vi "Set Ignition Data.vi"(8 "error in":errorcluster, 9 "result_ready":bool, 11 "Ignition in":refnum<class "Ignition.lvclass">) -> (0 "error out":errorcluster, 3 "Ignition out":refnum<class "Ignition.lvclass">)   [LabVIEW 2021, in "Ignition.lvclass"]
uses:
  Ignition.lvclass
  C:/GitHub/OOP_Submodule EOL/Sequence/CodeModules/OPC UA/OPC UA.lvclass
  OPC UA/OPC UA.lvclass/OPC UA.ctl
  Ignition.lvclass/Ignition.ctl
  <vilib>/addons/TestStand/_TSUtility.llb/TestStand - Get Property Value (Number {Signed 32-bit Integer}).vi
  <vilib>/addons/TestStand/_TSUtility.llb/TestStand - Get Property Value (String).vi
  <vilib>/addons/TestStand/_TSUtility.llb/TestStand - Get Property Value (Number {Unsigned 32-bit Integer}).vi
  <vilib>/addons/TestStand/_TSUtility.llb/TestStand - Get Property Value (Numeric Array).vi
  OPC UA/OPC UA.lvclass
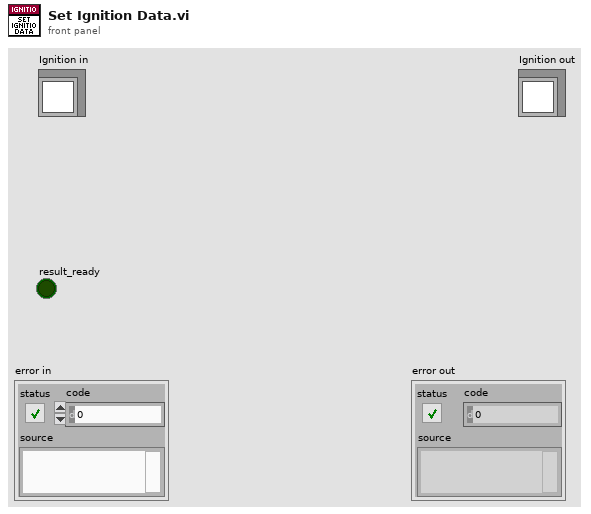
[diagram p1: front panel]
types:
  T1 = typedef "Ignition.lvclass/Tester Tx.ctl" = cluster{"thermistor":dbl, "phase_angle":dbl, "pallet_rfid":dbl, "ocv":dbl, "cell_vsense1":dbl, "cell_vsense2":dbl, "hipot1_leakage_current":dbl, "hipot2_leakage_current":dbl, "guid":string, "can_sn":string, "can_pn":string, "ac_internal_resistance":dbl, "sub_station":string, "fault_code":i32, "elapsed_time":i32, "result":i32, "reject_code_reason":string, "result_ready":bool, "Timeout":bool}
  T2 = cluster{"FaultCode":i32, "Fault codes":cluster{"Bit":string, "Description":string}[]}
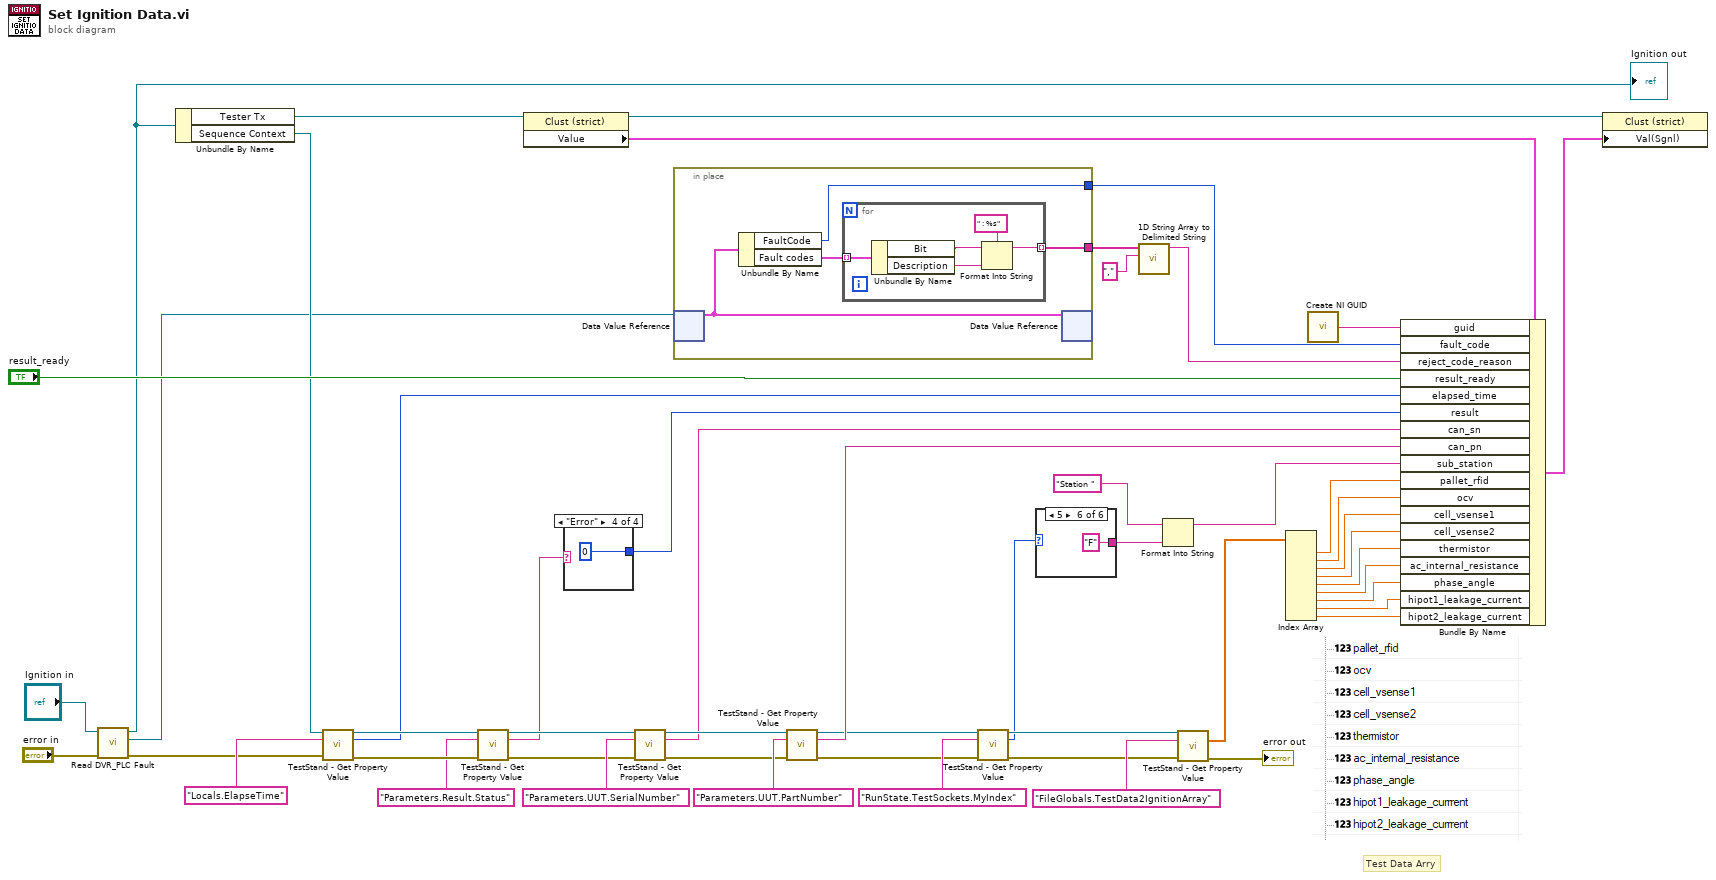
[diagram p0: block diagram]
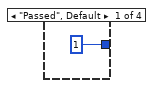
[diagram p2: hidden frame]
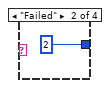
[diagram p3: hidden frame]
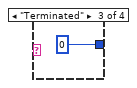
[diagram p4: hidden frame]
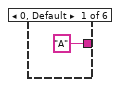
[diagram p5: hidden frame]
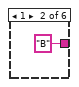
[diagram p6: hidden frame]
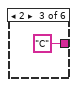
[diagram p7: hidden frame]
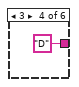
[diagram p8: hidden frame]
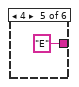
[diagram p9: hidden frame]
diagram:
  # "Test Data Arry"
  n1 = call "Read DVR_PLC Fault.vi"("error in (no error)"="error in", "OPC UA in"="Ignition in") -> ("error out"=w4:errorcluster, "DVR_PLC Fault"=w1:refnum<data-value>, "OPC UA out"=w2:refnum<class "Ignition.lvclass">)  [unwired: 7 in]
  "Ignition out" <- w2
  n2 = Unbundle By Name(w2) -> ("Tester Tx"=w13:refnum<vi>, "Sequence Context"=w14:refnum<k7>)
  n3 = call-poly <vilib>:"TestStand - Get Property Value.vi"("Sequence Context In"=w14, "Lookup String"="Locals.ElapseTime", "error in (no error)"=w4) -> ("Sequence Context Out"=w21:refnum<k7>, "Value"=w17:i32, "error out"=w23:errorcluster)  [unwired: 10 in]
  n4 = call-poly <vilib>:"TestStand - Get Property Value.vi"("Sequence Context In"=w21, "Lookup String"="Parameters.Result.Status", "error in (no error)"=w23) -> ("Sequence Context Out"=w20:refnum<k7>, "Value"=w16:string, "error out"=w19:errorcluster)  [unwired: 10 in]
  n5 = property class="Clust (strict)"(reference=w13) -> (reference out=w11:refnum<vi>, "Value"=w12:T1)  [unwired: 1 in, 1 out]
  n6 = case shown="\"Error\"" w16 {
    tunnel: [1 2 0 0] -> w15
    frame "Passed", Default {
    }
    frame "Failed" {
    }
    frame "Terminated" {
    }
    frame "Error" {
    }
  }
  n7 = call-poly <vilib>:"TestStand - Get Property Value.vi"("Sequence Context In"=w20, "Lookup String"="Parameters.UUT.SerialNumber", "error in (no error)"=w19) -> ("Sequence Context Out"=w51:refnum<k7>, "Value"=w48:string, "error out"=w49:errorcluster)  [unwired: 10 in]
  n8 = in-place {
    in-place-border: [w60] -> w9
    in-place-border: [w58] -> w6
    n9 = in-place-dvr #1(w1) -> (w59:T2)  [unwired: 1 out]
    n10 = Unbundle By Name(w59) -> ("FaultCode"=w58:i32, "Fault codes"=w57:cluster{"Bit":string, "Description":string}[])
    n11 = for {
      tunnel: w57 -> [w63] mode=indexing
      tunnel: [w64] -> w60 mode=indexing
      n12 = Unbundle By Name(w63) -> ("Bit"=w61:string, "Description"=w62:string)
      n13 = Format Into String(format string=" : %s", initial string=w61, w62) -> (resulting string=w64:string)  [unwired: 1 in, 1 out]
    }
    n14 = in-place-dvr #1(w59) -> ()  [unwired: 2 out]
  }
  n15 = call-poly <vilib>:"TestStand - Get Property Value.vi"("Sequence Context In"=w51, "Lookup String"="Parameters.UUT.PartNumber", "error in (no error)"=w49) -> ("Sequence Context Out"=w28:refnum<k7>, "Value"=w47:string, "error out"=w45:errorcluster)  [unwired: 10 in]
  n16 = call-poly <vilib>:"TestStand - Get Property Value.vi"("Sequence Context In"=w28, "Lookup String"="RunState.TestSockets.MyIndex", "error in (no error)"=w45) -> ("Sequence Context Out"=w43:refnum<k7>, "Value"=w27:u32, "error out"=w41:errorcluster)  [unwired: 10 in]
  n17 = case shown="5" w27 {
    tunnel: ["A" ("format string") "B" ("format string") "C" ("format string") "D" ("format string") "E" ("format string") "F" ("format string")] -> w26
    frame 0, Default {
    }
    frame 1 {
    }
    frame 2 {
    }
    frame 3 {
    }
    frame 4 {
    }
    frame 5 {
    }
  }
  n18 = call <vilib>:"1D String Array to Delimited String.vi"("delimiter"=",", "string array"=w9) -> ("delimited string"=w7:string)  [unwired: 9 in]
  n19 = Format Into String(initial string="Station ", w26) -> (resulting string=w44:string)  [unwired: 2 in, 1 out]
  n20 = call-poly <vilib>:"TestStand - Get Property Value.vi"("Sequence Context In"=w43, "Lookup String"="FileGlobals.TestData2IgnitionArray", "error in (no error)"=w41) -> ("Value"=w40:dbl[], "error out"=→"error out":errorcluster)  [unwired: 10 in, 1 out]
  n21 = Index Array(array=w40) -> (element #1=w39:dbl, element #2=w38:dbl, element #3=w37:dbl, element #4=w36:dbl, element #5=w35:dbl, element #6=w34:dbl, element #7=w33:dbl, element #8=w32:dbl, element #9=w31:dbl)  [unwired: 9 in]
  n22 = call <vilib>:"Create NI GUID.vi"() -> ("NI GUID"=w29:string)
  n23 = Bundle By Name(cluster=w12, "guid"=w29, "fault_code"=w6, "reject_code_reason"=w7, "result_ready"="result_ready", "elapsed_time"=w17, "result"=w15, "can_sn"=w48, "can_pn"=w47, "sub_station"=w44, "pallet_rfid"=w39, "ocv"=w38, "cell_vsense1"=w37, "cell_vsense2"=w36, "thermistor"=w35, "ac_internal_resistance"=w34, "phase_angle"=w33, "hipot1_leakage_current"=w32, "hipot2_leakage_current"=w31) -> (w10:T1)
  n24 = property class="Clust (strict)"(reference=w11, "Val(Sgnl)"=w10) -> ()  [unwired: 1 in, 2 out]
